vi "Write Collision Grid Info.vi"(8 "error in (no error)":errorcluster, 10 "Collision Grid Info":T1, 11 "Collider in":refnum<class "Collider.lvclass">) -> (0 "error out":errorcluster, 3 "Collider out":refnum<class "Collider.lvclass">)   [LabVIEW 2022 SP3, in "Collider.lvclass"]
uses:
  Collider.lvclass
  Collider.lvclass/Collider.ctl
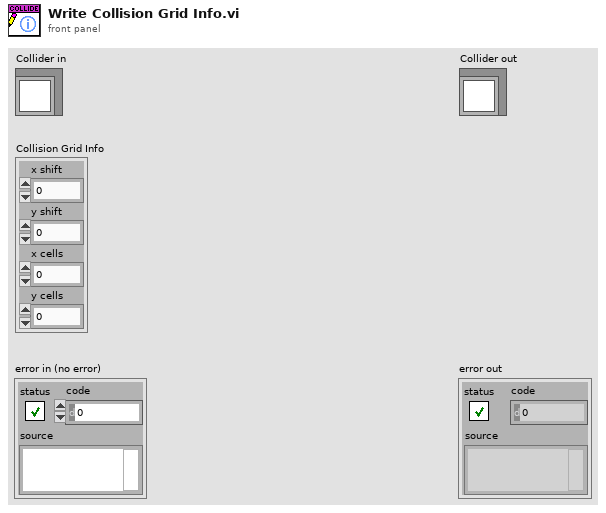
[diagram p1: front panel]
types:
  T1 = cluster{"x shift":i16, "y shift":i16, "x cells":i16, "y cells":i16}
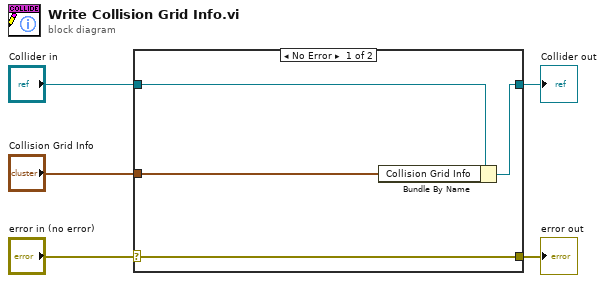
[diagram p0: block diagram]
diagram:
  n1 = case shown="No Error" "error in (no error)" {
    selector: "error in (no error)" -> [w9 w10]
    tunnel: [w9 w10] -> w4
    tunnel: [w7 w11] -> w2
    tunnel: "Collider in" -> [w8 w11]
    tunnel: "Collision Grid Info" -> [w6 _]
    frame No Error {
      n2 = Bundle By Name(cluster=w8, "Collision Grid Info"=w6) -> (w7:refnum<class "Collider.lvclass">)
    }
    frame Error {
    }
  }
  "error out" <- w4
  "Collider out" <- w2
